vi "DumbDash Get Tab Name.vi"(11 "Cluster":T1) -> (1 "Rest of Name":string, 3 "Tab Name":string)   [LabVIEW 2017]
uses:
  DumbDash Control.ctl
  DumbDash Control Type.ctl
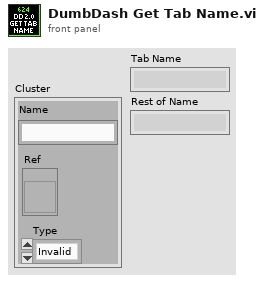
[diagram p1: front panel]
types:
  T1 = typedef "DumbDash Control.ctl" = cluster{"Name":string, "Ref":refnum<vi>, "Type":T2}
  T2 = typedef "DumbDash Control Type.ctl" = enum16{"Invalid", "Number", "Boolean", "String"}
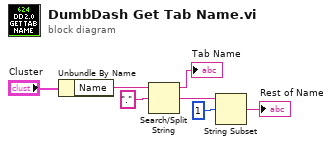
[diagram p0: block diagram]
diagram:
  n1 = Unbundle By Name("Cluster") -> ("Name"=w6:string)
  n2 = Search/Split String(string=w6, search string/char (-)=".") -> (substring before match=→"Tab Name":string, match + rest of string=w3:string)  [unwired: 1 in, 1 out]
  n3 = String Subset(string=w3, offset (0)=1) -> (substring=→"Rest of Name":string)  [unwired: 1 in]
